vi "Motor position to frequency.vi"(10 "Fit parameters":cluster{"Slope":dbl, "Intercept":dbl}, 11 "Motor position":dbl) -> (3 "Frequency":dbl)   [LabVIEW 2015]
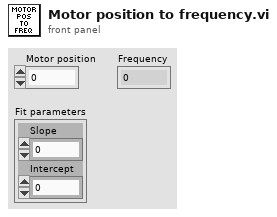
[diagram p1: front panel]
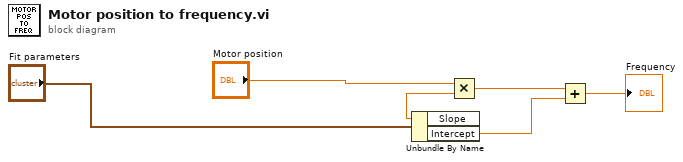
[diagram p0: block diagram]
diagram:
  n1 = Unbundle By Name("Fit parameters") -> ("Slope"=w3:dbl, "Intercept"=w6:dbl)
  n2 = Multiply(x="Motor position", y=w3) -> (x*y=w5:dbl)
  n3 = Add(x=w5, y=w6) -> (x+y=→"Frequency":dbl)
